vi "main.vi"() -> ()   [LabVIEW 2023]
uses:
  CONTROLS/states.ctl
panel:
  out "Meldung":string
  out "Enum 2":T1
  in  "stop":bool
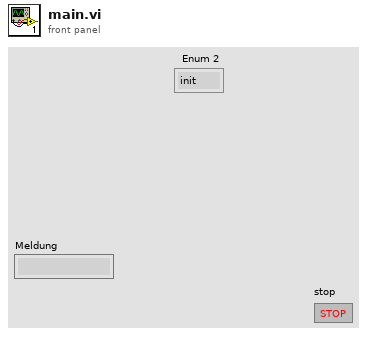
[diagram p1: front panel]
types:
  T1 = typedef "states.ctl" = enum16{"init", "read", "write", "Kundeneingabe", "Betonauswahl", "Bezahlprozess", "Rechnung", "Zutaten mit Gewichtmessung", "Stop"}
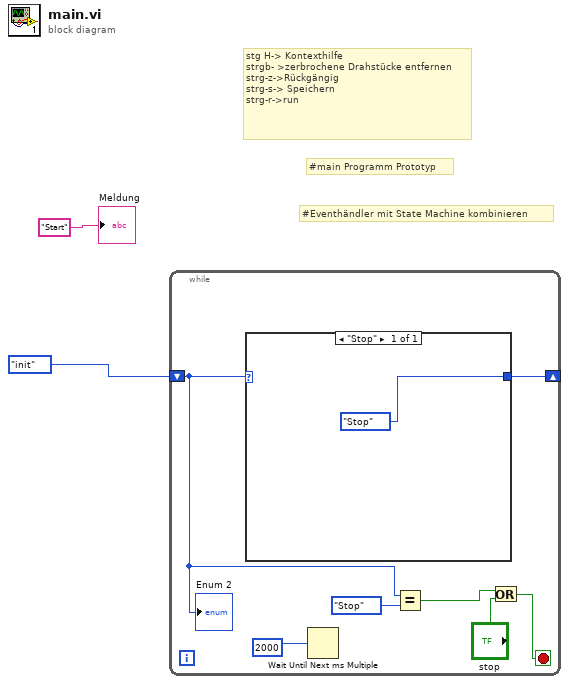
[diagram p0: block diagram]
diagram:
  # "#Eventhändler mit State Machine kombinieren"
  # "#main Programm Prototyp"
  # "stg H-> Kontexthilfe\nstrgb- >zerbrochene Drahstücke entfernen\nstrg-z->Rückgängig\nstrg-s-> Speichern\nstrg-r->run"
  n1 = while {
    shift-right: [w9] -> _
    shift-left: states."init" -> [w4]
    stop <- w7 stop-if-true
    n2 = case shown="\"Stop\"" w4 {
      tunnel: [states."Stop"] -> w9
      frame "Stop" {
      }
    }
    n3 = Wait Until Next ms Multiple(millisecond multiple=2000) -> ()  [unwired: 1 out]
    n4 = Equal?(x=w4, y=states."Stop") -> (x = y?=w5:bool)
    n5 = Or(x=w5, y="stop") -> (x .or. y?=w7:bool)
    "Enum 2" <- w4
  }
  "Meldung" <- "Start"
